vi "Configure DC Monitor.vi"(8 "error in (no error)":errorcluster, 9 "Current DC Monitor State (T:Enable)":bool=TRUE, 10 "Voltage DC Monitor State (T:Enable)":bool=TRUE, 11 "VISA resource name":refnum<visa-resource-name>) -> (0 "error out":errorcluster, 3 "VISA resource name out":refnum<visa-resource-name>)   [LabVIEW 2017, in "Agilent E4980.lvlib"]
doc: "Enables or disables the DC voltage level and the DC current level monitor.\n\n<B>Notes:</B>\n(1) This is valid only when your instrument installs <B>Option 001</B> (Power and DC Bias enhancement)."
uses:
  Agilent E4980.lvlib
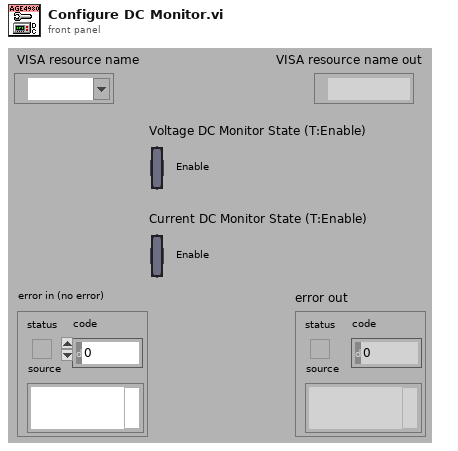
[diagram p1: front panel]
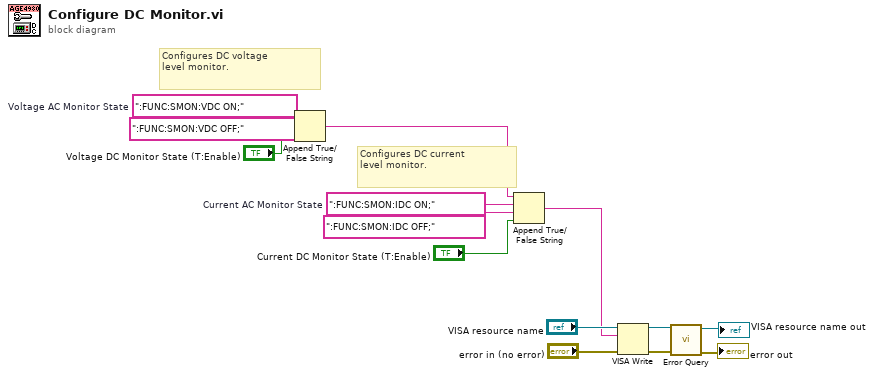
[diagram p0: block diagram]
diagram:
  w1 = ":FUNC:SMON:IDC ON;"  # Current AC Monitor State
  w12 = ":FUNC:SMON:VDC ON;"  # Voltage AC Monitor State
  # "Configures DC voltage\nlevel monitor."
  # "Configures DC current\nlevel monitor."
  n1 = Append True/False String(1:"Voltage DC Monitor State (T:Enable)", 2:":FUNC:SMON:VDC OFF;" ("false string"), 3:w12) -> (0:w11:string)  [unwired: 1 in]
  n2 = Append True/False String(1:"Current DC Monitor State (T:Enable)", 2:":FUNC:SMON:IDC OFF;", 3:w1, 4:w11) -> (0:w6:string)
  n3 = VISA Write(VISA resource name="VISA resource name", write buffer=w6, error in (no error)="error in (no error)") -> (VISA resource name out=w5:refnum<visa-resource-name>, error out=w4:errorcluster)  [unwired: 1 out]
  n4 = call "Error Query.vi"("error in (no error)"=w4, "VISA resource name"=w5) -> ("error out"=→"error out":errorcluster, "VISA resource name out"=→"VISA resource name out":refnum<visa-resource-name>)  [unwired: 6 in, 2 out]
